vi "NI-XNET Monitor Async.vi"(10 "Parameters":variant, 11 "Process":refnum<class "Process.lvclass">) -> ()   [LabVIEW 2018, in "NI-XNET Monitor Engine.lvlib"]
uses:
  NI-XNET Monitor Engine.lvlib
  <vilib>/NI/NIVS Inline Async API/_VS Inline Async API/Process/Process.lvclass
  <vilib>/NI/NIVS Inline Async API/_VS Inline Async API/Process/Process.lvclass/Process.ctl
  <vilib>/NI/NIVS Inline Async API/_VS Inline Async API/Process/Data Member Access/Read Data Access.vi
  <vilib>/NI/NIVS Inline Async API/_VS Inline Async API/Error Handling Process/SubVIs/Error.ConvertArray.vi
  <vilib>/NI/NIVS Inline Async API/_Data Access Engine/Data Access Engine/Data Access Engine.lvclass
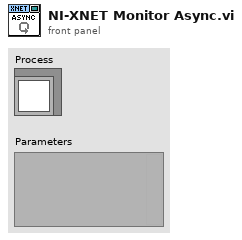
[diagram p1: front panel]
types:
  T1 = typedef "NI-XNET Monitor Engine.lvlib/RTMonitorRefnums.ctl" = cluster{"CAN":cluster{"Session":refnum<k21>, "ChN Ref":T2}[], "FlexRay":cluster{"Session":refnum<k21>, "ChN Ref":T2}[], "LIN":cluster{"Session":refnum<k21>, "ChN Ref":T2}[]}
  T2 = typedef "Data Access Engine.lvlib/Data Access Engine.lvclass/Write.DVR.ctl" = refnum<data-value>
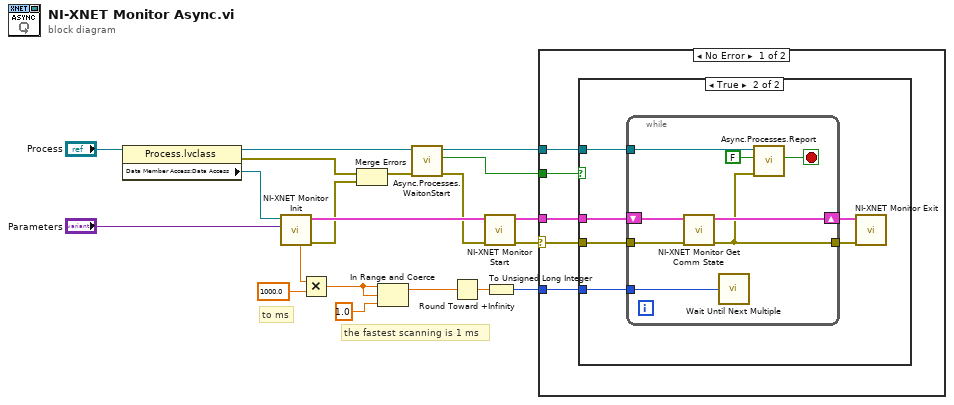
[diagram p0: block diagram]
diagram:
  # "the fastest scanning is 1 ms"
  # "to ms"
  n1 = property class="Process.lvclass"(reference="Process") -> (reference out=w17:refnum<class "Process.lvclass">, error out=w14:errorcluster, "Data Member Access:Data Access"=w15:refnum<class "Data Access Engine.lvclass">)  [unwired: 1 in]
  n2 = call "NI-XNET Monitor Init.vi"("Parameters"="Parameters", "Data Access Engine in"=w15) -> ("Error Out"=w10:errorcluster, "Process  Data Out"=w13:T1, "Async Loop Rate (s)"=w7:dbl)  [unwired: 7 in]
  n3 = Multiply(x=w7, y=1000.0) -> (x*y=w4:dbl)
  n4 = Merge Errors(w14, w10) -> (w2:errorcluster)
  n5 = In Range and Coerce(upper limit=w4, x=w4, lower limit=1.0) -> (coerced(x)=w6:dbl)  [unwired: 1 out]
  n6 = call <vilib>:"Async.Processes.WaitonStart.vi"("error in (no error)"=w2, "Process"=w17) -> ("error out"=w11:errorcluster, "Execute"=w20:bool, "Process out"=w19:refnum<class "Process.lvclass">)  [unwired: 7 in]
  n7 = Round Toward +Infinity(x=w6) -> (ceil(x): smallest int >= x=w8:dbl)
  n8 = call "NI-XNET Monitor Start.vi"("Error In"=w11, "Process  Data In"=w13) -> ("Error Out"=w1:errorcluster, "Process  Data Out"=w12:T1)  [unwired: 8 in]
  n9 = To Unsigned Long Integer(number=w8) -> (unsigned 32bit integer=w9:u32)
  n10 = case shown="No Error" w1 {
    selector: w1 -> [w23 _]
    tunnel: w20 -> [w25 _]
    tunnel: w19 -> [w24 _]
    tunnel: w12 -> [w22 _]
    tunnel: w9 -> [w21 _]
    frame No Error {
      n11 = case shown="True" w25 {
        tunnel: w24 -> [_ w30]
        tunnel: w23 -> [_ w29]
        tunnel: w22 -> [_ w31]
        tunnel: w21 -> [_ w26]
        frame False {
        }
        frame True {
          n12 = while {
            tunnel: w30 -> [w33]
            tunnel: w29 -> [w35]
            shift-right: [w38] -> w28
            shift-left: w31 -> [w37]
            tunnel: [w34] -> w27
            tunnel: w26 -> [w32]
            stop <- w39 stop-if-true
            n13 = call "NI-XNET Monitor Get Comm State.vi"("Error In"=w35, "Process  Data In"=w37) -> ("Error Out"=w34:errorcluster, "Process  Data Out"=w38:T1)  [unwired: 8 in]
            n14 = call "Wait Until Next Multiple"("Count(mSec)"=w32) -> ()  [unwired: 1 out]
            n15 = call <vilib>:"Async.Processes.Report.vi"("Error"=w34, "Stop Async on Error?"=FALSE ("Stop on Error?"), "Process in"=w33) -> ("Stop"=w39:bool)  [unwired: 7 in, 1 out]
          }
          n16 = call "NI-XNET Monitor Exit.vi"("Error In"=w27, "Process  Data In"=w28) -> ()  [unwired: 8 in, 2 out]
        }
      }
    }
    frame Error {
    }
  }
